vi "CAN STP Engine Tx Data FGV.vi"(6 "CAN FGV State":T1=enum."Get", 8 "error in":errorcluster, 10 "Socket No":i16, 11 "STP Engine Tx Data in":refnum<queue>) -> (0 "error out":errorcluster, 2 "STP Engine Tx Data Array":refnum<queue>[](array[refnum]), 3 "STP Engine Tx Data out":refnum<queue>)   [LabVIEW 2023, in "LTT_TeststandSteptypes.lvlib"]
uses:
  LTT_TeststandSteptypes.lvlib
  Control/CAN FGV State.ctl
  STP Engine SubVI/Control/STP Engine Tx Data.ctl
  HardwareAbstractionLayer_LVOOP/CAN/CAN Application Protocols/STP Protocol_class/Ctrls/STP Input Data.ctl
  HardwareAbstractionLayer_LVOOP/CAN/CAN Application Protocols/STP Protocol_class/Ctrls/STP CMD.ctl
  HardwareAbstractionLayer_LVOOP/CAN/CAN Application Protocols/STP Protocol_class/STP Protocol.lvclass
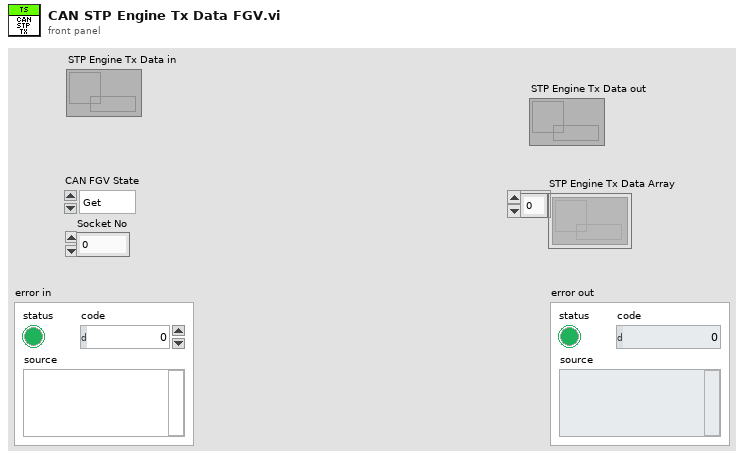
[diagram p1: front panel]
types:
  T1 = typedef "LTT_TeststandSteptypes.lvlib/CAN FGV State.ctl" = enum16{"Init", "Get", "Set"}
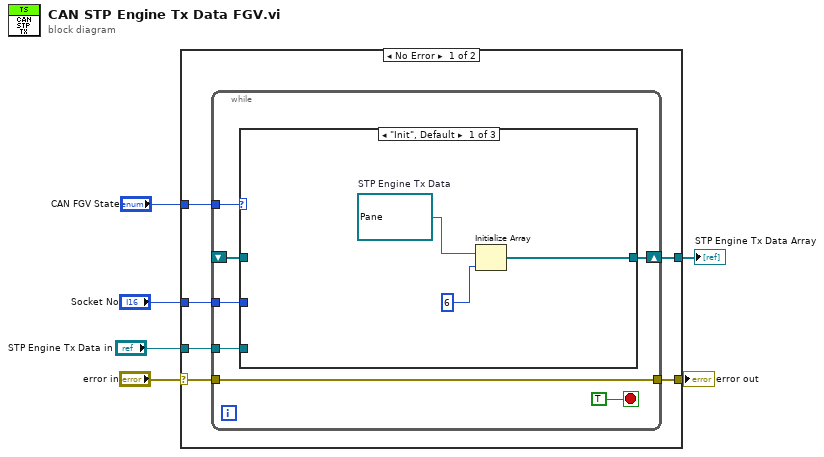
[diagram p0: block diagram]
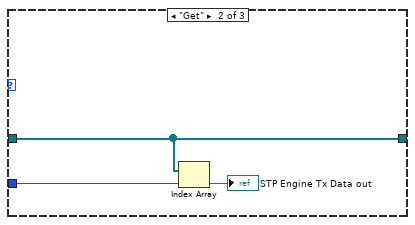
[diagram p2: hidden frame]
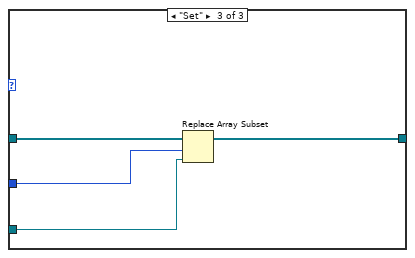
[diagram p3: hidden frame]
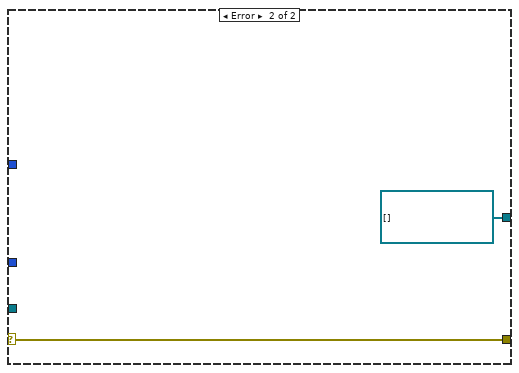
[diagram p4: hidden frame]
diagram:
  n1 = case shown="No Error" "error in" {
    selector: "error in" -> [w12 w31]
    tunnel: "CAN FGV State" -> [w11 _]
    tunnel: "Socket No" -> [w10 _]
    tunnel: [w9 w31] -> w3
    tunnel: [w8 refnum<queue>[] []] -> w2
    tunnel: "STP Engine Tx Data in" -> [w7 _]
    frame No Error {
      n2 = while {
        tunnel: w12 -> [w14]
        tunnel: w11 -> [w18]
        shift-right: [w17] -> w8
        shift-left: _ -> [w16]
        tunnel: w10 -> [w15]
        tunnel: [w14] -> w9
        tunnel: w7 -> [w13]
        stop <- TRUE stop-if-true
        n3 = case shown="\"Init\", Default" w18 {
          tunnel: [w22 w24 w28] -> w17
          tunnel: w16 -> [_ w24 w29]
          tunnel: w15 -> [_ w25 w27]
          tunnel: w13 -> [_ _ w26]
          frame "Init", Default {
            w20 = refnum<queue> refnum  # STP Engine Tx Data
            n4 = Initialize Array(w20, 6 ("dimension size")) -> (w22:refnum<queue>[])
          }
          frame "Get" {
            n5 = Index Array(array=w24, index=w25) -> (element=→"STP Engine Tx Data out":refnum<queue>)
          }
          frame "Set" {
            n6 = Replace Array Subset(array=w29, new element=w26, index=w27) -> (w28:refnum<queue>[])
          }
        }
      }
    }
    frame Error {
    }
  }
  "error out" <- w3
  "STP Engine Tx Data Array" <- w2
